vi "Insert Open VI.vi"(8 "error in":errorcluster, 10 "Replacement VI":path, 11 "Destination VI":path) -> (0 "error out":errorcluster)   [LabVIEW 2014]
uses:
  <vilib>/Utility/VariantDataType/Type.ctl
  <vilib>/Utility/traverseref.llb/TRef TravTarget.ctl
  <vilib>/Utility/traverseref.llb/VI Scripting - Traverse.lvlib
  <vilib>/Utility/VariantDataType/VariantType.lvlib
panel:
  out "Contains Data Type to Find?":bool
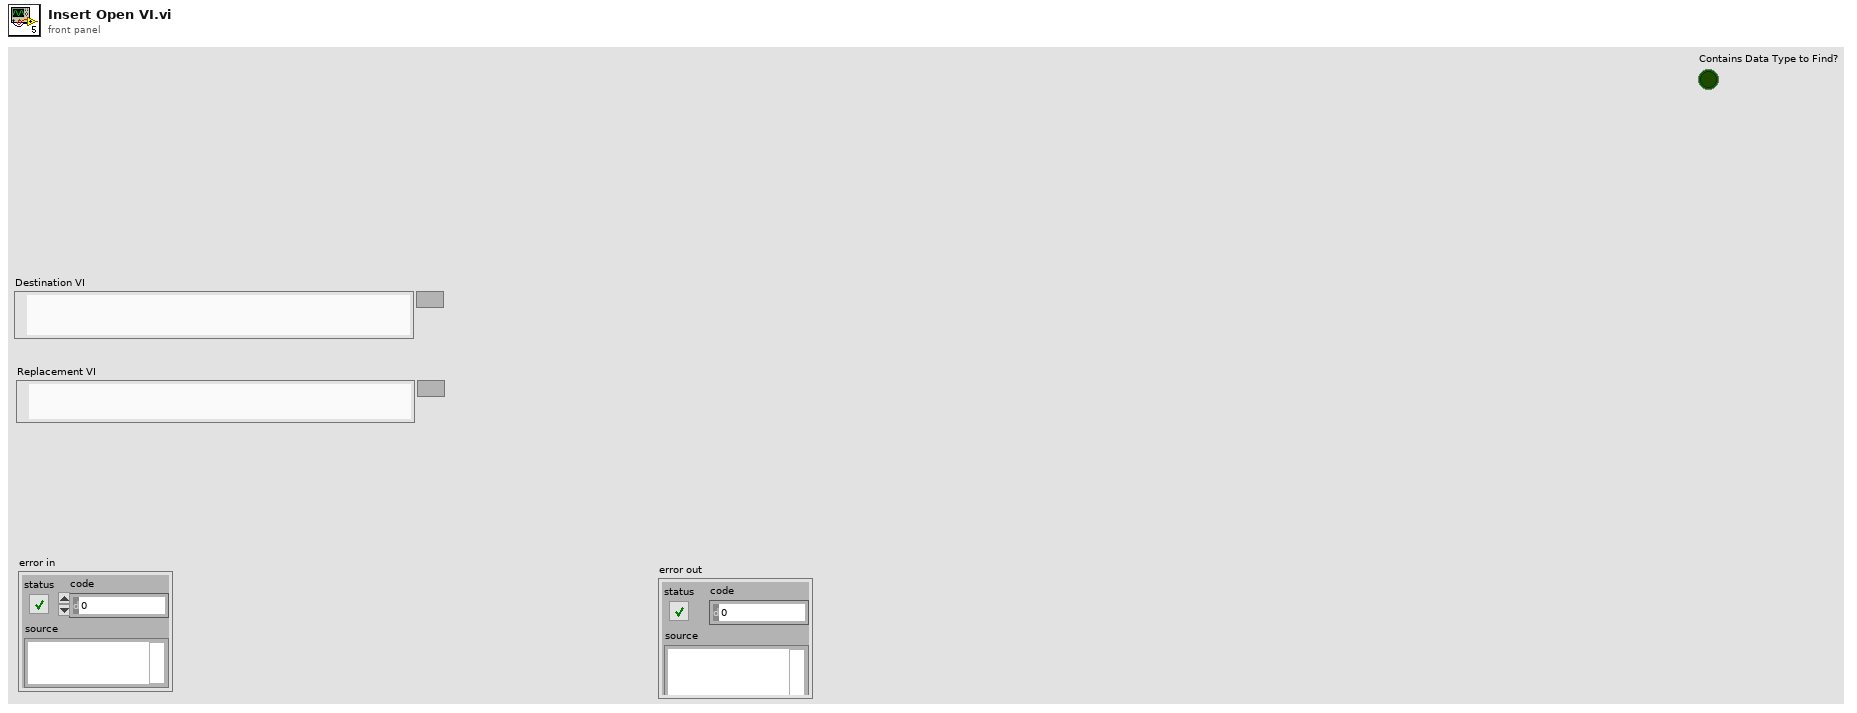
[diagram p1: front panel]
types:
  T1 = typedef "VariantType.lvlib/Type.ctl" = enum8{"Invalid Type", "Void", "I8", "I16", "I32", "I64", "U8", "U16", "U32", "U64", "Single Float", "Double Float", "Extended Float", "Single Complex", "Double Complex", "Extended Complex", "Enum U8", "Enum U16", "Enum U32", "Enum U64", "Single Float With Unit", "Double Float With Unit", "Extended Float With Unit", "Single Complex with Unit", "Double Complex with Unit", "Extended Complex with Unit", "Boolean", "String", "Path", "Picture", "Tag", "Array", "Cluster", "Variant", "LV Variant", "Waveform", "Timestamp", "Digital Waveform", "Digital Data", "ExpressData", "Refnum", "External Data", "VI", "Poly VI", "LabVIEW Class Instance", "Fixed Point"}
  T2 = typedef "TRef TravTarget.ctl" = enum16{"FP", "BD", "Other"}
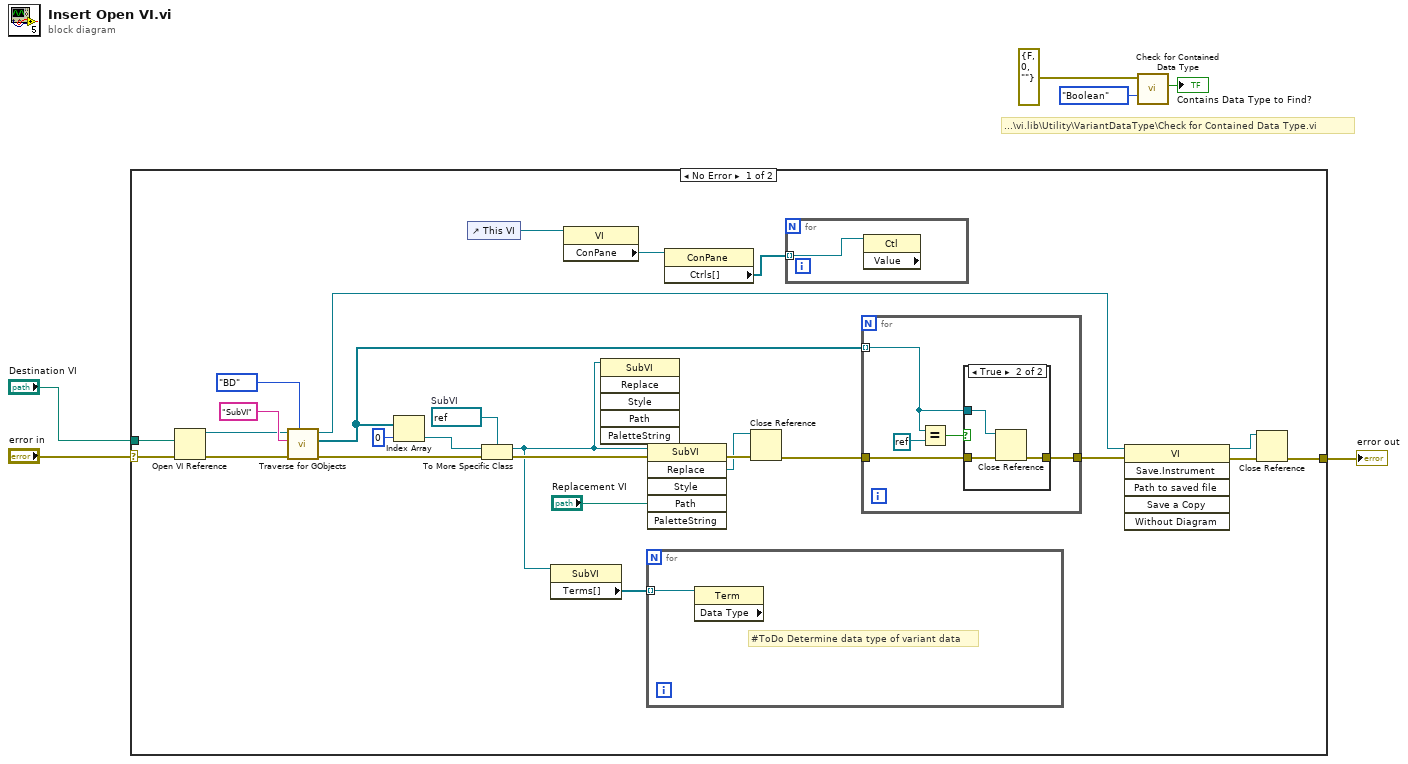
[diagram p0: block diagram]
diagram:
  # "...\\vi.lib\\Utility\\VariantDataType\\Check for Contained Data Type.vi"
  n1 = case shown="No Error" "error in" {
    selector: "error in" -> [w24 w44]
    tunnel: [w27 w44] -> w5
    tunnel: "Destination VI" -> [w21 _]
    frame No Error {
      w20 = refnum<vi> refnum  # SubVI
      n2 = Open VI Reference(vi path=w21, error in (no error)=w24) -> (vi reference=w22:refnum<vi>, error out=w23:errorcluster)  [unwired: 4 in]
      n3 = call <vilib>:"Traverse for GObjects.vi"("Traverse Target"=TRef_TravTarget."BD", "error in (no error)"=w23, "Class Name"="SubVI", "VI Refnum"=w22) -> ("error out"=w17:errorcluster, "References"=w19:refnum<vi>[], "dup VI Refnum"=w28:refnum<vi>)  [unwired: 4 in, 1 out]
      n4 = Index Array(array=w19, index=0) -> (element=w11:refnum<vi>)
      n5 = control-ref of="This VI"() -> (w9:refnum<vi>)
      n6 = To More Specific Class(target class=w20, reference=w11, error in=w17) -> (specific class reference=w10:refnum<vi>, error out=w13:errorcluster)
      n7 = property class="SubVI"(reference=w10) -> ("Terms[]"=w12:refnum<vi>[])  [unwired: 1 in, 2 out]
      n8 = property class="VI"(reference=w9) -> ("ConPane"=w8:refnum<vi>)  [unwired: 1 in, 2 out]
      n9 = invoke class="SubVI" method="Replace"(reference=w10) -> ()  [unwired: 5 in, 6 out]
      n10 = for {
        tunnel: w12 -> [w34] mode=indexing
        # "#ToDo Determine data type of variant data"
        n11 = property class="Term" props=["Data Type"](reference=w34) -> ()  [unwired: 1 in, 3 out]
      }
      n12 = invoke class="SubVI" method="Replace"(reference=w10, error in=w13, "Path"="Replacement VI") -> (error out=w15:errorcluster, "Replace"=w14:refnum<vi>)  [unwired: 3 in, 4 out]
      n13 = property class="ConPane"(reference=w8) -> ("Ctrls[]"=w7:refnum<vi>[])  [unwired: 1 in, 2 out]
      n14 = Close Reference(reference=w14, error in (no error)=w15) -> (error out=w30:errorcluster)
      n15 = for {
        tunnel: w7 -> [w33] mode=indexing
        n16 = property class="Ctl" props=["Value"](reference=w33) -> ()  [unwired: 1 in, 3 out]
      }
      n17 = for {
        tunnel: w30 -> [w39]
        tunnel: [w38] -> w29
        tunnel: w19 -> [w35] mode=indexing
        n18 = Equal?(x=w35, y=refnum<k0> refnum) -> (x = y?=w36:bool)
        n19 = case shown="True" w36 {
          tunnel: w39 -> [w40 w43]
          tunnel: [w40 w42] -> w38
          tunnel: w35 -> [_ w41]
          frame False {
          }
          frame True {
            n20 = Close Reference(reference=w41, error in (no error)=w43) -> (error out=w42:errorcluster)
          }
        }
      }
      n21 = invoke class="VI" method="Save.Instrument"(reference=w28, error in=w29) -> (reference out=w25:refnum<vi>, error out=w26:errorcluster)  [unwired: 4 in, 4 out]
      n22 = Close Reference(reference=w25, error in (no error)=w26) -> (error out=w27:errorcluster)
    }
    frame Error {
    }
  }
  "error out" <- w5
  n23 = call <vilib>:"Check for Contained Data Type.vi"("Data Type to Find"=Type."Boolean", "Data Type"=errorcluster {"status"=FALSE, "code"=0, "source"=""} ("error out")) -> ("Contains Data Type to Find?"=→"Contains Data Type to Find?":bool)  [unwired: 7 in, 2 out]
